vi "SubVI_ReadFile_Auto.vi"(9 "file path (dialog if empty)":path=path "C:/Users/Public/Documents/Howdybots/2018NewPowerUpHB/AutoScripts/test.csv") -> (1 "subarray":string[](array[string]))   [LabVIEW 2017]
uses:
  <vilib>/Utility/file.llb/Read Delimited Spreadsheet (string).vi
  <vilib>/Rock Robotics/Network Tables/NT Write String Array.vi
panel:
  out "first row":string[](array[string])
  out "all rows":string[][](array[string])
  in  "delimiter (,)":string
  in  "error in":errorcluster
  out "error out":errorcluster
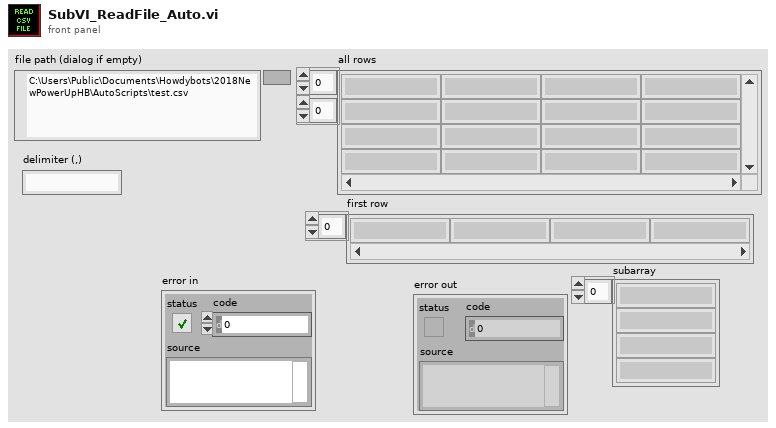
[diagram p1: front panel]
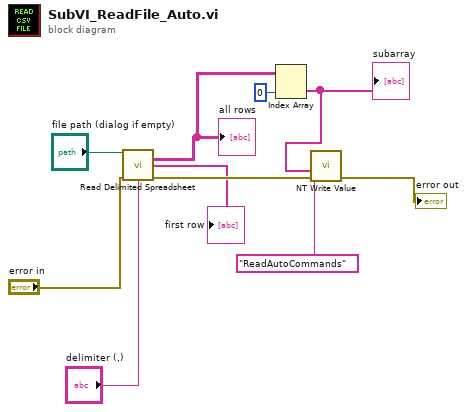
[diagram p0: block diagram]
diagram:
  n1 = call-poly <vilib>:"Read Delimited Spreadsheet.vi"("file path (dialog if empty)"="file path (dialog if empty)", "error in (no error)"="error in", "delimiter (\\t)"="delimiter (,)") -> ("all rows"=w4:string[][], "first row"=→"first row":string[], "error out"=→"error out":errorcluster)  [unwired: 7 in, 3 out]
  "all rows" <- w4
  n2 = Index Array(array=w4, index (col)=0 ("disabled index (col)")) -> (element=w2:string[])  [unwired: 1 in]
  "subarray" <- w2
  n3 = call-poly <vilib>:"NT Write Value.vi"("String Array"=w2, "Name"="ReadAutoCommands") -> ()  [unwired: 9 in, 1 out]
